vi "Fetch Scope Records.vi"(8 "error in (no error)":errorcluster, 11 "Panel State Data In":T2) -> (0 "error out":errorcluster, 2 "Captured Waveforms":T1(graph), 3 "Panel State Data Out":T2)   [LabVIEW 2025]
uses:
  Typedef/Test Panel State Data.ctl
  <instrlib>/niScope/Acquire/Fetch/niScope Multi Fetch.vi
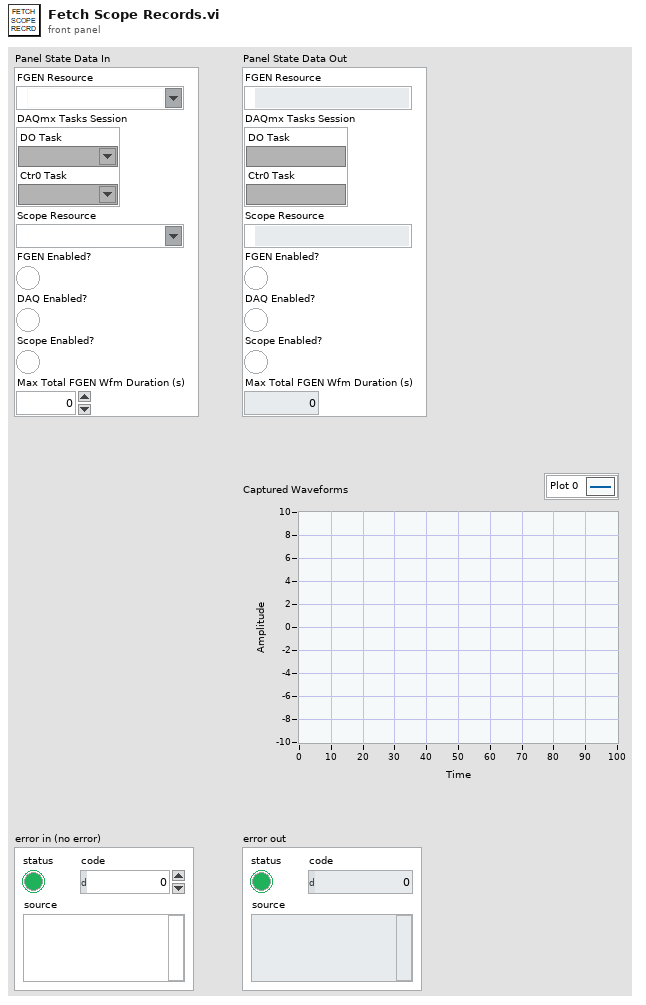
[diagram p1: front panel]
types:
  T1 = cluster{"relativeInitialX":dbl, "xIncrement":dbl, "wfm":dbl[]}[]
  T2 = typedef "Test Panel State Data.ctl" = cluster{"FGEN Resource":refnum<k15>, "DAQmx Tasks Session":cluster{"DO Task":refnum<k21>, "Ctr0 Task":refnum<k21>}, "Scope Resource":refnum<k15>, "FGEN Enabled?":bool, "DAQ Enabled?":bool, "Scope Enabled?":bool, "Max Total FGEN Wfm Duration (s)":dbl}
  T3 = cluster{"actualSamples":i32, "absoluteInitialX":dbl, "relativeInitialX":dbl, "xIncrement":dbl, "offset":dbl, "gain":dbl, "reserved1":dbl, "reserved2":dbl}[]
  T4 = cluster{"relativeInitialX":dbl, "xIncrement":dbl, "wfm":dbl[]}
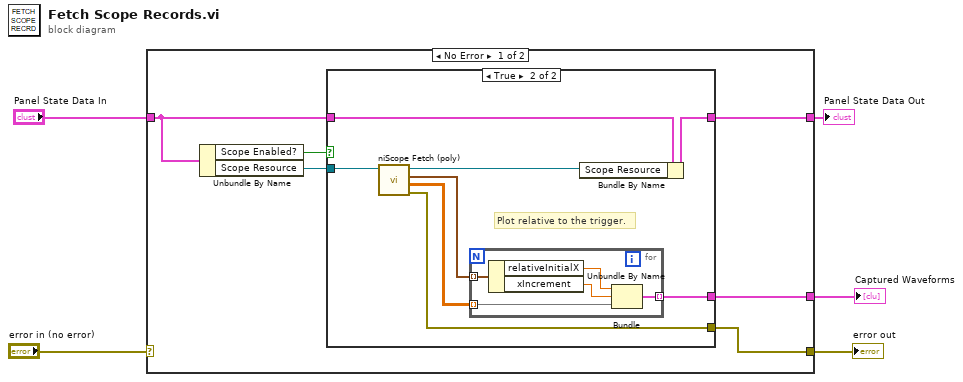
[diagram p0: block diagram]
diagram:
  n1 = case shown="No Error" "error in (no error)" {
    selector: "error in (no error)" -> [_ w27]
    tunnel: "Panel State Data In" -> [w11 w26]
    tunnel: [w6 w27] -> w5
    tunnel: [w10 w26] -> w2
    tunnel: [w7 _] -> w1
    frame No Error {
      n2 = Unbundle By Name(w11) -> ("Scope Enabled?"=w9:bool, "Scope Resource"=w8:refnum<k15>)
      n3 = case shown="True" w9 {
        tunnel: w11 -> [w12 w20]
        tunnel: [w12 w19] -> w10
        tunnel: w8 -> [_ w18]
        tunnel: [_ w14] -> w7
        tunnel: [_ w13] -> w6
        frame False {
        }
        frame True {
          # "Plot relative to the trigger."
          n4 = call-poly <instrlib>:"niScope Fetch (poly).vi"("instrument handle"=w18) -> ("error out"=w13:errorcluster, "wfm"=w15:dbl[][], "wfm info"=w16:T3, "instrument handle out"=w17:refnum<k15>)  [unwired: 7 in]
          n5 = for {
            tunnel: w15 -> [w23] mode=indexing
            tunnel: [w22] -> w14 mode=indexing
            tunnel: w16 -> [w21] mode=indexing
            n6 = Unbundle By Name(w21) -> ("relativeInitialX"=w25:dbl, "xIncrement"=w24:dbl)
            n7 = Bundle("relativeInitialX"=w25, "xIncrement"=w24, "wfm"=w23) -> (w22:T4)  [unwired: 1 in]
          }
          n8 = Bundle By Name(cluster=w20, "Scope Resource"=w17) -> (w19:T2)
        }
      }
    }
    frame Error {
    }
  }
  "error out" <- w5
  "Panel State Data Out" <- w2
  "Captured Waveforms" <- w1
